vi "Run.vi"(8 "error in (no error)":errorcluster, 11 "socket REP in":refnum<class "socket REP.lvclass">) -> (0 "error out":errorcluster, 3 "socket REP out":refnum<class "socket REP.lvclass">)   [LabVIEW 2018, in "socket REP.lvclass"]
uses:
  socket REP.lvclass
  C:/Users/orlando/Documents/Orlando/communication-manager/communication-manager/Socket/Socket.lvclass
  Socket/Socket.lvclass
  State Machine/State Machine.lvclass
  RxTx/RxTx.lvclass
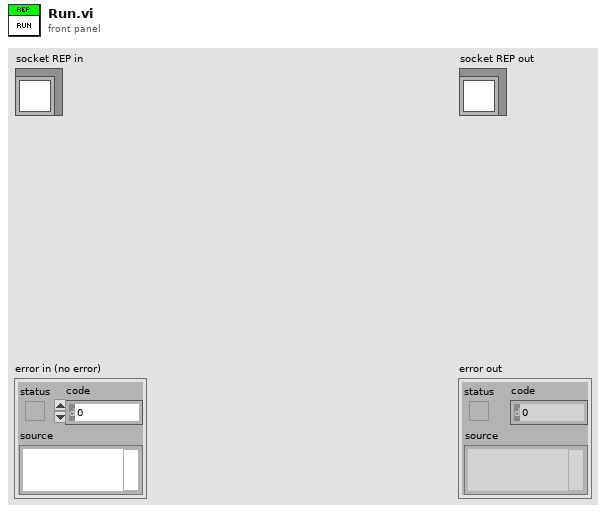
[diagram p1: front panel]
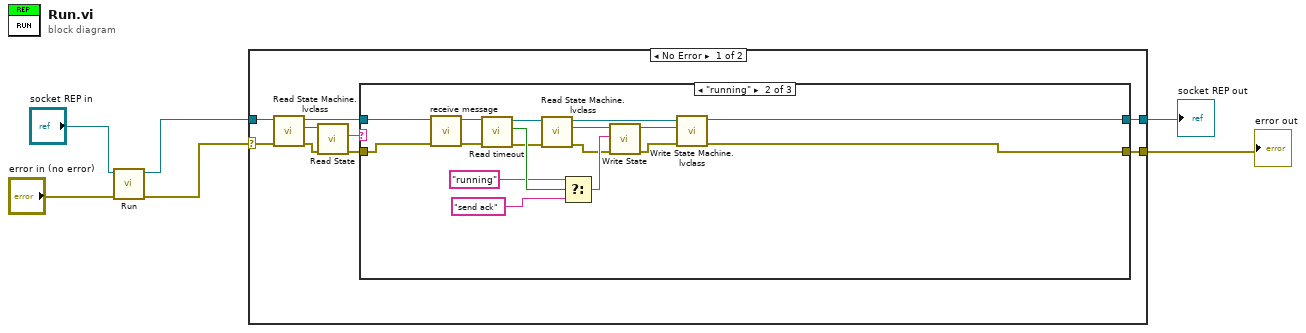
[diagram p0: block diagram]
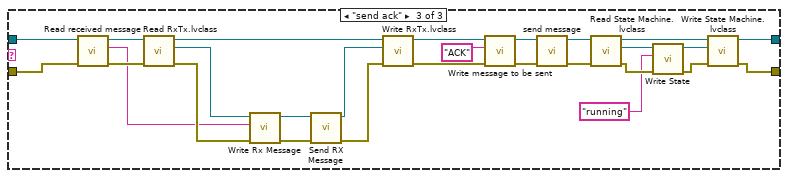
[diagram p3: hidden frame]
diagram:
  n1 = call-parent "Run.vi"("error in (no error)"="error in (no error)", "Socket in"="socket REP in") -> ("error out"=w3:errorcluster, "Socket out"=w4:refnum<class "socket REP.lvclass">)  [unwired: 8 in]
  n2 = case shown="No Error" w3 {
    selector: w3 -> [w9 w61]
    tunnel: w4 -> [w10 w62]
    tunnel: [w13 w62] -> w1
    tunnel: [w14 w61] -> w2
    frame No Error {
      n3 = call-dynamic "Read State Machine.lvclass.vi"("error in (no error)"=w9, "Socket in"=w10) -> ("error out"=w8:errorcluster, "State Machine.lvclass"=w11:refnum<class "State Machine.lvclass">, "Socket out"=w7:refnum<class "socket REP.lvclass">)  [unwired: 7 in]
      n4 = call-dynamic "Read State.vi"("error in (no error)"=w8, "State Machine in"=w11) -> ("error out"=w12:errorcluster, "State"=w15:string)  [unwired: 7 in, 1 out]
      n5 = case shown="\"running\"" w15 {
        tunnel: [w16 w18 w35] -> w13
        tunnel: [w17 w19 w36] -> w14
        tunnel: w12 -> [w17 w33 w46]
        tunnel: w7 -> [w16 w34 w45]
        frame Default {
        }
        frame "running" {
          n6 = call-dynamic "receive message.vi"("error in (no error)"=w33, "Socket in"=w34) -> ("error out"=w31:errorcluster, "Socket out"=w32:refnum<class "socket REP.lvclass">)  [unwired: 8 in]
          n7 = call-dynamic "Read timeout.vi"("error in (no error)"=w31, "Socket in"=w32) -> ("error out"=w25:errorcluster, "timeout"=w30:bool, "Socket out"=w26:refnum<class "socket REP.lvclass">)  [unwired: 7 in]
          n8 = call-dynamic "Read State Machine.lvclass.vi"("error in (no error)"=w25, "Socket in"=w26) -> ("error out"=w24:errorcluster, "State Machine.lvclass"=w22:refnum<class "State Machine.lvclass">, "Socket out"=w20:refnum<class "socket REP.lvclass">)  [unwired: 7 in]
          n9 = Select(t="running", s=w30, f="send ack") -> (s? t:f=w28:string)
          n10 = call-dynamic "Write State.vi"("error in (no error)"=w24, "State"=w28, "State Machine in"=w22) -> ("error out"=w23:errorcluster, "State Machine out"=w21:refnum<class "State Machine.lvclass">)  [unwired: 7 in]
          n11 = call-dynamic "Write State Machine.lvclass.vi"("error in (no error)"=w23, "State Machine.lvclass"=w21, "Socket in"=w20) -> ("error out"=w19:errorcluster, "Socket out"=w18:refnum<class "socket REP.lvclass">)  [unwired: 7 in]
        }
        frame "send ack" {
          n12 = call-dynamic "Read received message.vi"("error in (no error)"=w46, "Socket in"=w45) -> ("error out"=w56:errorcluster, "received message"=w55:string, "Socket out"=w52:refnum<class "socket REP.lvclass">)  [unwired: 7 in]
          n13 = call-dynamic "Read RxTx.lvclass.vi"("Socket in"=w52) -> ("RxTx.lvclass"=w53:refnum<class "RxTx.lvclass">, "Socket out"=w50:refnum<class "socket REP.lvclass">)  [unwired: 8 in, 1 out]
          n14 = call "Write Rx Message.vi"("error in (no error)"=w56, "Rx Message"=w55, "RxTx in"=w53) -> ("error out"=w54:errorcluster, "RxTx out"=w57:refnum<class "RxTx.lvclass">)  [unwired: 7 in]
          n15 = call "Send RX Message.vi"("error in (no error)"=w54, "RxTx in"=w57) -> ("error out"=w49:errorcluster, "RxTx out"=w51:refnum<class "RxTx.lvclass">)  [unwired: 8 in]
          n16 = call-dynamic "Write RxTx.lvclass.vi"("error in (no error)"=w49, "RxTx.lvclass"=w51, "Socket in"=w50) -> ("error out"=w48:errorcluster, "Socket out"=w47:refnum<class "socket REP.lvclass">)  [unwired: 7 in]
          n17 = call-dynamic "Write message to be sent.vi"("error in (no error)"=w48, "message to be sent"="ACK", "Socket in"=w47) -> ("error out"=w59:errorcluster, "Socket out"=w60:refnum<class "socket REP.lvclass">)  [unwired: 7 in]
          n18 = call "send message.vi"("error in (no error)"=w59, "Socket in"=w60) -> ("error out"=w38:errorcluster, "Socket out"=w37:refnum<class "socket REP.lvclass">)  [unwired: 8 in]
          n19 = call-dynamic "Read State Machine.lvclass.vi"("error in (no error)"=w38, "Socket in"=w37) -> ("error out"=w44:errorcluster, "State Machine.lvclass"=w42:refnum<class "State Machine.lvclass">, "Socket out"=w40:refnum<class "socket REP.lvclass">)  [unwired: 7 in]
          n20 = call-dynamic "Write State.vi"("error in (no error)"=w44, "State"="running", "State Machine in"=w42) -> ("error out"=w43:errorcluster, "State Machine out"=w41:refnum<class "State Machine.lvclass">)  [unwired: 7 in]
          n21 = call-dynamic "Write State Machine.lvclass.vi"("error in (no error)"=w43, "State Machine.lvclass"=w41, "Socket in"=w40) -> ("error out"=w36:errorcluster, "Socket out"=w35:refnum<class "socket REP.lvclass">)  [unwired: 7 in]
        }
      }
    }
    frame Error {
    }
  }
  "error out" <- w2
  "socket REP out" <- w1
